vi "Get Control Value.vi"(8 "error in (no error)":errorcluster, 9 "label":string, 10 "object class":T1, 11 "Panel":refnum<vi>) -> (0 "error out":errorcluster, 1 "value":variant, 3 "Panel out":refnum<vi>)   [LabVIEW 2018, in "NISAST VI Scripting.lvlib" / "VI.lvlib" / "Front Panel.lvlib"]
uses:
  Front Panel.lvlib
  Type Define/Object Class.ctl
  Agilent N5232A PNA-L/Labview Driver/Keysight PNA Series/express/Utility/StudioHelper/Common/VI Scripting/Type Define/Type Define.lvlib
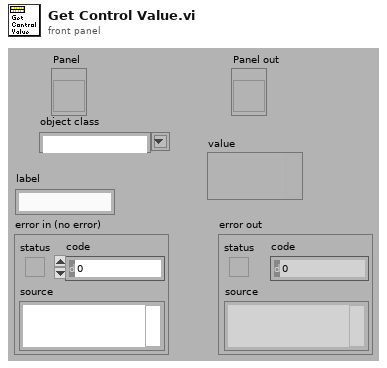
[diagram p1: front panel]
types:
  T1 = typedef "NISAST VI Scripting.lvlib/Type Define.lvlib/Object Class.ctl" = string
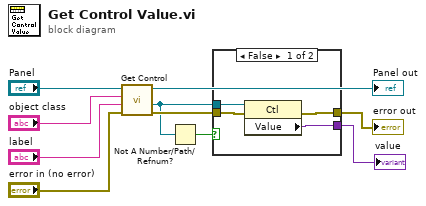
[diagram p0: block diagram]
diagram:
  n1 = call "Get Control.vi"("error in (no error)"="error in (no error)", "label"="label", "object class"="object class", "Panel"="Panel") -> ("error out"=w8:errorcluster, "first control"=w2:refnum<vi>, "Panel out"=→"Panel out":refnum<vi>)  [unwired: 5 out]
  n2 = Not A Number/Path/Refnum?(number/path/refnum=w2) -> (NaN/Path/Refnum?=w3:bool)
  n3 = case shown="False" w3 {
    tunnel: w8 -> [w14 w15]
    tunnel: [w13 w15] -> w5
    tunnel: [w12 _] -> w4
    tunnel: w2 -> [w11 _]
    frame False {
      n4 = property class="Ctl"(reference=w11, error in=w14) -> (error out=w13:errorcluster, "Value"=w12:variant)  [unwired: 1 out]
    }
    frame True {
    }
  }
  "value" <- w4
  "error out" <- w5
